vi "x_y_graph_cluster_solar_array_sim.vi"(1 "Chart History (10,000)":i32, 2 "Clear Graph?":bool, 3 "X":dbl, 4 "Y":dbl) -> (0 "Cluster":cluster{dbl[], dbl[]})   [LabVIEW 2016]
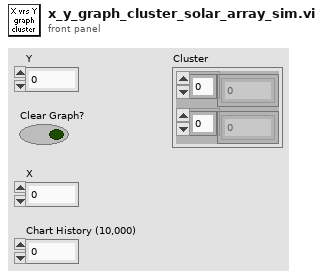
[diagram p1: front panel]
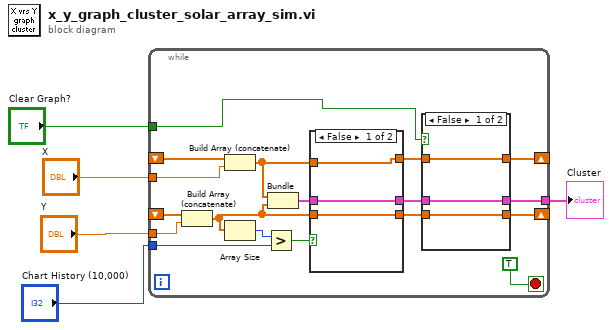
[diagram p0: block diagram]
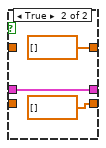
[diagram p2: hidden frame]
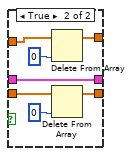
[diagram p3: hidden frame]
diagram:
  n1 = while {
    tunnel: "X" -> [w23]
    tunnel: "Y" -> [w21]
    shift-right: [w10] -> _
    shift-left: _ -> [w22]
    shift-right: [w13] -> _
    shift-left: _ -> [w20]
    tunnel: "Chart History (10,000)" -> [w18]
    tunnel: [w8] -> w3
    tunnel: "Clear Graph?" -> [w6]
    stop <- TRUE stop-if-true
    n2 = Build Array (concatenate)(w20, w21) -> (w15:dbl[])
    n3 = Build Array (concatenate)(w22, w23) -> (w12:dbl[])
    n4 = Array Size(array=w15) -> (size(s)=w19:i32)
    n5 = Greater?(x=w19, y=w18) -> (0:w17:bool)
    n6 = Bundle(w12, w15) -> (w16:cluster{dbl[], dbl[]})  [unwired: 1 in]
    n7 = case shown="False" w17 {
      tunnel: w16 -> [w30 w33]
      tunnel: w15 -> [w32 w35]
      tunnel: [w32 w34] -> w14
      tunnel: [w31 w38] -> w11
      tunnel: w12 -> [w31 w39]
      tunnel: [w30 w33] -> w9
      frame False {
      }
      frame True {
        n8 = Delete From Array(array=w39, index=0) -> (array with subset deleted=w38:dbl[])  [unwired: 1 in, 1 out]
        n9 = Delete From Array(array=w35, index=0) -> (array with subset deleted=w34:dbl[])  [unwired: 1 in, 1 out]
      }
    }
    n10 = case shown="False" w6 {
      tunnel: w14 -> [w26 _]
      tunnel: [w26 dbl[] []] -> w13
      tunnel: w11 -> [w25 _]
      tunnel: [w25 dbl[] []] -> w10
      tunnel: [w24 w27] -> w8
      tunnel: w9 -> [w24 w27]
      frame False {
      }
      frame True {
      }
    }
  }
  "Cluster" <- w3
